vi "Weather Parse Test.vi"() -> ()   [LabVIEW 2020, in "CDM-Config.lvlib"]
uses:
  CDM-Config.lvlib
  <vilib>/httpClient/LabVIEWHTTPClient.lvlib
  Config-JSON/Config-JSON.lvclass
  Config Manager/Config Manager.lvclass
panel:
  out "error out":errorcluster
  in  "Tree":string(tree)
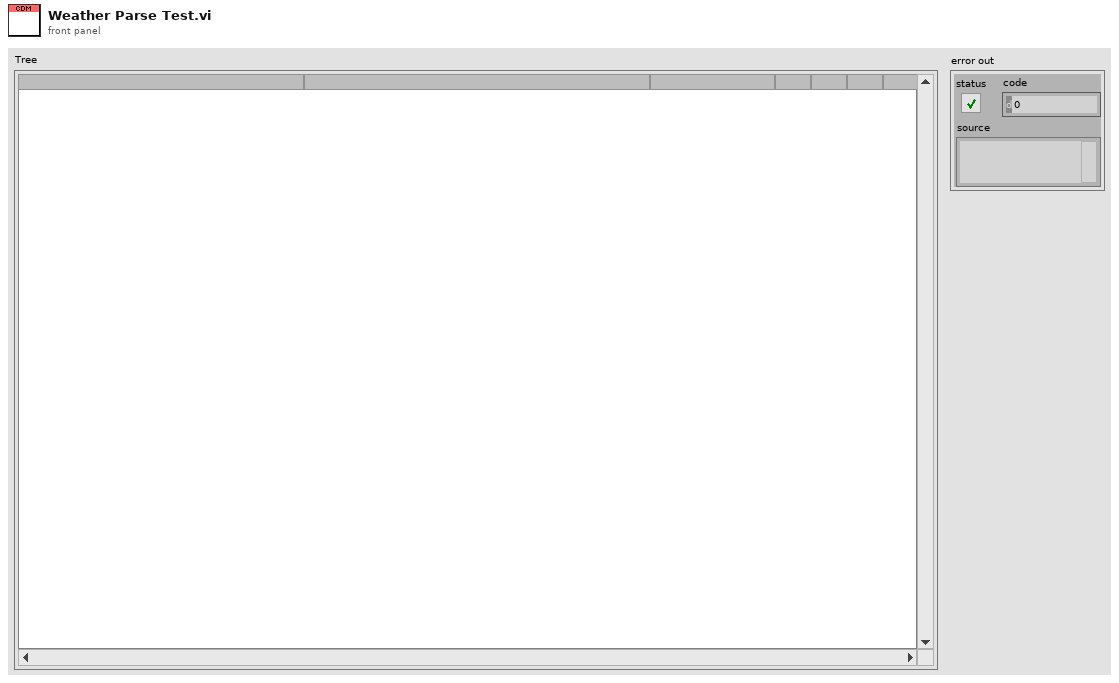
[diagram p1: front panel]
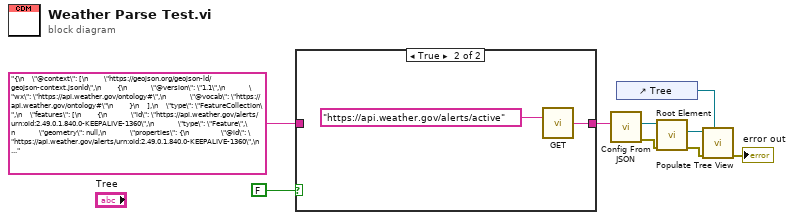
[diagram p0: block diagram]
diagram:
  n1 = case shown="True" FALSE {
    tunnel: [w10 w11] -> w7
    tunnel: "{\n    \"@context\": [\n        \"https://geojson.org/geojson-ld/geojson-context.jsonld\",\n        {\n            \"@version\": \"1.1\",\n            \"wx\": \"https://api.weather.gov/ontology#\",\n            \"@vocab\": \"https://api.weather.gov/ontology#\"\n        }\n    ],\n    \"type\": \"FeatureCollection\",\n    \"features\": [\n        {\n            \"id\": \"https://api.weather.gov/alerts/urn:oid:2.49.0.1.840.0-KEEPALIVE-1360\",\n            \"type\": \"Feature\",\n            \"geometry\": null,\n            \"properties\": {\n                \"@id\": \"https://api.weather.gov/alerts/urn:oid:2.49.0.1.840.0-KEEPALIVE-1360\",\n                \"@type\": \"wx:Alert\",\n                \"id\": \"urn:oid:2.49.0.1.840.0-KEEPALIVE-1360\",\n                \"areaDesc\": \"Montgomery\",\n                \"geocode\": {\n                    \"SAME\": [\n                        \"024031\"\n                    ],\n                    \"UGC\": [\n                        \"MDC031\"\n                    ]\n                },\n                \"affectedZones\": [\n                    \"https://api.weather.gov/zones/county/MDC031\"\n                ],\n                \"references\": [],\n                \"sent\": \"2025-12-03T16:14:45+00:00\",\n                \"effective\": \"2025-12-03T16:14:45+00:00\",\n                \"onset\": null,\n                \"expires\": \"2025-12-03T16:24:45+00:00\",\n                \"ends\": null,\n                \"status\": \"Test\",\n                \"messageType\": \"Alert\",\n                \"category\": \"Met\",\n                \"severity\": \"Unknown\",\n                \"certainty\": \"Unknown\",\n                \"urgency\": \"Unknown\",\n                \"event\": \"Test Message\",\n                \"sender\": \"w-nws.webmaster@noaa.gov\",\n                \"senderName\": \"NWS\",\n                \"headline\": null,\n                \"description\": \"Monitoring message only. Please disregard.\",\n                \"instruction\": \"Monitoring message only. Please disregard.\",\n                \"response\": \"None\",\n                \"parameters\": {\n                    \"AWIPSidentifier\": [\n                        \"KEPWBC\"\n                    ],\n                    \"WMOidentifier\": [\n                        \"NZUS91 KWBC 031614\"\n                    ],\n                    \"BLOCKCHANNEL\": [\n                        \"CMAS\",\n                        \"EAS\",\n                        \"NWEM\"\n                    ]\n                },\n                \"scope\": \"Public\",\n                \"code\": \"IPAWSv1.0\",\n                \"language\": \"en-US\",\n                \"web\": \"http://www.weather.gov\",\n                \"eventCode\": {\n                    \"SAME\": [\n                        \"NWS\"\n                    ],\n                    \"NationalWeatherService\": [\n                        \"TST\"\n                    ]\n                }\n            }\n        },\n        {\n            \"id\": \"https://api.weather.gov/alerts/urn:oid:2.49.0.1.840.0.cd44bbbaaabdcac51418f4171d6c2d57f83e8e62.002.1\",\n            \"type\": \"Feature\",\n            \"geometry\": null,\n            \"properties\": {\n                \"@id\": \"https://api.weather.gov/alerts/urn:oid:2.49.0.1.840.0.cd44bbbaaabdcac51418f4171d6c2d57f83e8e62.002.1\",\n                \"@type\": \"wx:Alert\",\n                \"id\": \"urn:oid:2.49.0.1.840.0.cd44bbbaaabdcac51418f4171d6c2d57f83e8e62.002.1\",\n                \"areaDesc\": \"Lake Michigan from Seul Choix Point to Rock Island Passage 5NM offshore to Mid Lake; Lake Michigan South of a line from Seul Choix Point to the Mackinac Bridge and North of a line from Charlevoix MI to South Fox Island 5NM offshore; Lake Michigan from Charlevoix to Point Betsie MI 5NM Offshore to mid lake; Lake Michigan from Point Betsie to Manistee MI 5NM offshore to Mid Lake; Lake Michigan from Rock Island Passage to Sturgeon Bay WI 5NM offshore to mid lake; Lake Michigan from Sturgeon Bay to Two Rivers WI 5NM offshore to Mid Lake\",\n                \"geocode\": {\n                    \"SAME\": [\n                        \"092261\",\n                        \"092362\",\n                        \"092364\",\n                        \"092366\",\n                        \"092563\",\n                        \"092565\"\n                    ],\n                    \"UGC\": [\n                        \"LMZ261\",\n                        \"LMZ362\",\n                        \"LMZ364\",\n                        \"LMZ366\",\n                        \"LMZ563\",\n                        \"LMZ565\"\n                    ]\n                },\n                \"affectedZones\": [\n                    \"https://api.weather.gov/zones/forecast/LMZ261\",\n                    \"https://api.weather.gov/zones/forecast/LMZ362\",\n                    \"https://api.weather.gov/zones/forecast/LMZ364\",\n                    \"https://api.weather.gov/zones/forecast/LMZ366\",\n                    \"https://api.weather.gov/zones/forecast/LMZ563\",\n                    \"https://api.weather.gov/zones/forecast/LMZ565\"\n                ],\n                \"references\": [\n                    {\n                        \"@id\": \"https://api.weather.gov/alerts/urn:oid:2.49.0.1.840.0.87140d8193f69fdde7a236498f0c417a3c416cc9.002.1\",\n                        \"identifier\": \"urn:oid:2.49.0.1.840.0.87140d8193f69fdde7a236498f0c417a3c416cc9.002.1\",\n                        \"sender\": \"w-nws.webmaster@noaa.gov\",\n                        \"sent\": \"2025-12-03T01:49:00-06:00\"\n                    }\n                ],\n                \"sent\": \"2025-12-03T10:07:00-06:00\",\n                \"effective\": \"2025-12-03T10:07:00-06:00\",\n                \"onset\": \"2025-12-04T21:00:00-06:00\",\n                \"expires\": \"2025-12-03T18:15:00-06:00\",\n                \"ends\": \"2025-12-05T06:00:00-06:00\",\n                \"status\": \"Actual\",\n                \"messageType\": \"Update\",\n                \"category\": \"Met\",\n                \"severity\": \"Moderate\",\n                \"certainty\": \"Possible\",\n                \"urgency\": \"Future\",\n                \"event\": \"Gale Watch\",\n                \"sender\": \"w-nws.webmaster@noaa.gov\",\n                \"senderName\": \"NWS Milwaukee/Sullivan WI\",\n                \"headline\": \"Gale Watch issued December 3 at 10:07AM CST until December 5 at 6:00AM CST by NWS Milwaukee/Sullivan WI\",\n                \"description\": \"* WHAT...Southwest winds 20 to 30 kt with gusts up to 40 kt and\\nwaves 7 to 12 ft possible.\\n\\n* WHERE...Northern Third of the Open Waters of Lake Michigan,\\nLake Michigan from Point Betsie to Manistee MI 5NM offshore to\\nMid Lake, and Lake Michigan from Sturgeon Bay to Two Rivers WI\\n5NM offshore to Mid Lake.\\n\\n* WHEN...From Thursday evening through late Thursday night.\\n\\n* IMPACTS...Strong winds can cause hazardous waves which could\\ncapsize or damage vessels and reduce visibility.\",\n                \"instruction\": \"Mariners should consider altering plans to avoid possible\\nhazardous conditions.  Remain in port, seek safe harbor, alter\\ncourse, and/or secure the vessel for severe wind and waves.\",\n                \"response\": \"Prepare\",\n                \"parameters\": {\n                    \"AWIPSidentifier\": [\n                        \"MWWMKX\"\n                    ],\n                    \"WMOidentifier\": [\n                        \"WHUS73 KMKX 031607\"\n                    ],\n                    \"NWSheadline\": [\n                        \"GALE WATCH REMAINS IN EFFECT FROM THURSDAY EVENING THROUGH LATE THURSDAY NIGHT\"\n                    ],\n                    \"BLOCKCHANNEL\": [\n                        \"EAS\",\n                        \"NWEM\",\n                        \"CMAS\"\n                    ],\n                    \"VTEC\": [\n                        \"/O.CON.KMKX.GL.A.0026.251205T0300Z-251205T1200Z/\"\n                    ],\n                    \"eventEndingTime\": [\n                        \"2025-12-05T06:00:00-06:00\"\n                    ]\n                },\n                \"scope\": \"Public\",\n                \"code\": \"IPAWSv1.0\",\n                \"language\": \"en-US\",\n                \"web\": \"http://www.weather.gov\",\n                \"eventCode\": {\n                    \"SAME\": [\n                        \"NWS\"\n                    ],\n                    \"NationalWeatherService\": [\n                        \"GLA\"\n                    ]\n                }\n            }\n        },\n        {\n            \"id\": \"https://api.weather.gov/alerts/urn:oid:2.49.0.1.840.0.cd44bbbaaabdcac51418f4171d6c2d57f83e8e62.001.1\",\n            \"type\": \"Feature\",\n            \"geometry\": null,\n            \"properties\": {\n                \"@id\": \"https://api.weather.gov/alerts/urn:oid:2.49.0.1.840.0.cd44bbbaaabdcac51418f4171d6c2d57f83e8e62.001.1\",\n                \"@type\": \"wx:Alert\",\n                \"id\": \"urn:oid:2.49.0.1.840.0.cd44bbbaaabdcac51418f4171d6c2d57f83e8e62.001.1\",\n                \"areaDesc\": \"Sheboygan to Port Washington WI; Port Washington to North Point Light WI; North Point Light to Wind Point WI; Wind Point WI to Winthrop Harbor IL\",\n                \"geocode\": {\n                    \"SAME\": [\n                        \"092643\",\n                        \"092644\",\n                        \"092645\",\n                        \"092646\"\n                    ],\n                    \"UGC\": [\n                        \"LMZ643\",\n                        \"LMZ644\",\n                        \"LMZ645\",\n                        \"LMZ646\"\n                    ]\n                },\n                \"affectedZones\": [\n                    \"https://api.weather.gov/zones/forecast/LMZ643\",\n                    \"https://api.weather.gov/zones/forecast/LMZ644\",\n                    \"https://api.weather.gov/zones/forecast/LMZ645\",\n                    \"https://api.weather.gov/zones/forecast/LMZ646\"\n                ],\n                \"references\": [\n                    {\n                        \"@id\": \"https://api.weather.gov/alerts/urn:oid:2.49.0.1.840.0.87140d8193f69fdde7a236498f0c417a3c416cc9.001.1\",\n                        \"identifier\": \"urn:oid:2.49.0.1.840.0.87140d8193f69fdde7a236498f0c417a3c416cc9.001.1\",\n                        \"sender\": \"w-nws.webmaster@noaa.gov\",\n                        \"sent\": \"2025-12-03T01:49:00-06:00\"\n                    }\n                ],\n                \"sent\": \"2025-12-03T10:07:00-06:00\",\n                \"effective\": \"2025-12-03T10:07:00-06:00\",\n                \"onset\": \"2025-12-03T10:07:00-06:00\",\n                \"expires\": \"2025-12-03T18:15:00-06:00\",\n                \"ends\": \"2025-12-04T06:00:00-06:00\",\n                \"status\": \"Actual\",\n                \"messageType\": \"Update\",\n                \"category\": \"Met\",\n                \"severity\": \"Minor\",\n                \"certainty\": \"Likely\",\n                \"urgency\": \"Expected\",\n                \"event\": \"Small Craft Advisory\",\n                \"sender\": \"w-nws.webmaster@noaa.gov\",\n                \"senderName\": \"NWS Milwaukee/Sullivan WI\",\n                \"headline\": \"Small Craft Advisory issued December 3 at 10:07AM CST until December 4 at 6:00AM CST by NWS Milwaukee/Sullivan WI\",\n                \"description\": \"* WHAT...Northwest winds 15 to 20 kt with gusts up to 25 kt.\\n\\n* WHERE...Nearshore Waters from Sheboygan to Winthrop Harbor IL.\\n\\n* WHEN...Until 6 AM CST Thursday.\\n\\n* IMPACTS...Conditions will be hazardous to small craft.\",\n                \"instruction\": \"Inexperienced mariners, especially those operating smaller\\nvessels, should avoid navigating in hazardous conditions.\",\n                \"response\": \"Avoid\",\n                \"parameters\": {\n                    \"AWIPSidentifier\": [\n                        \"MWWMKX\"\n                    ],\n                    \"WMOidentifier\": [\n                        \"WHUS73 KMKX 031607\"\n                    ],\n                    \"NWSheadline\": [\n                        \"SMALL CRAFT ADVISORY REMAINS IN EFFECT UNTIL 6 AM CST THURSDAY\"\n                    ],\n                    \"BLOCKCHANNEL\": [\n                        \"EAS\",\n                        \"NWEM\",\n                        \"CMAS\"\n                    ],\n                    \"VTEC\": [\n                        \"/O.CON.KMKX.SC.Y.0105.000000T0000Z-251204T1200Z/\"\n                    ],\n                    \"eventEndingTime\": [\n                        \"2025-12-04T06:00:00-06:00\"\n                    ],\n                    \"expiredReferences\": [\n                        \"w-nws.webmaster@noaa.gov,urn:oid:2.49.0.1.840.0.8bd0308a1f57db3dacad4c3397c13ff936336f9a.001.1,2025-12-02T20:55:00-06:00 w-nws.webmaster@noaa.gov,urn:oid:2.49.0.1.840.0.6281cc536b0e67be3da54b18c0c55c2862a1bde1.001.1,2025-12-02T14:15:00-06:00 w-nws.webmaster@noaa.gov,urn:oid:2.49.0.1.840.0.2f172b9f18f65013fb5f156b8abb524ff0d234b7.001.1,2025-12-02T08:57:00-06:00 w-nws.webmaster@noaa.gov,urn:oid:2.49.0.1.840.0.b1896b6562e7fd8378f844b86b23eedf120466cc.001.1,2025-12-02T02:26:00-06:00\"\n                    ]\n                },\n                \"scope\": \"Public\",\n                \"code\": \"IPAWSv1.0\",\n                \"language\": \"en-US\",\n                \"web\": \"http://www.weather.gov\",\n                \"eventCode\": {\n                    \"SAME\": [\n                        \"NWS\"\n                    ],\n                    \"NationalWeatherService\": [\n                        \"SCY\"\n                    ]\n                }\n            }\n        },\n        {\n            \"id\": \"https://api.weather.gov/alerts/urn:oid:2.49.0.1.840.0.cfec64fd36b2ac790d0ebe73b8c20f8dfc3ec5cb.007.1\",\n            \"type\": \"Feature\",\n            \"geometry\": null,\n            \"properties\": {\n                \"@id\": \"https://api.weather.gov/alerts/urn:oid:2.49.0.1.840.0.cfec64fd36b2ac790d0ebe73b8c20f8dfc3ec5cb.007.1\",\n                \"@type\": \"wx:Alert\",\n                \"id\": \"urn:oid:2.49.0.1.840.0.cfec64fd36b2ac790d0ebe73b8c20f8dfc3ec5cb.007.1\",\n                \"areaDesc\": \"Saxon Harbor WI to Black River MI\",\n                \"geocode\": {\n                    \"SAME\": [\n                        \"091240\"\n                    ],\n                    \"UGC\": [\n                        \"LSZ240\"\n                    ]\n                },\n                \"affectedZones\": [\n                    \"https://api.weather.gov/zones/forecast/LSZ240\"\n                ],\n                \"references\": [\n                    {\n                        \"@id\": \"https://api.weather.gov/alerts/urn:oid:2.49.0.1.840.0.e016f252f56054b547b3ac73b3419f6e51da412e.009.1\",\n                        \"identifier\": \"urn:oid:2.49.0.1.840.0.e016f252f56054b547b3ac73b3419f6e51da412e.009.1\",\n                        \"sender\": \"w-nws.webmaster@noaa.gov\",\n                        \"sent\": \"2025-12-03T03:23:00-05:00\"\n                    }\n                ],\n                \"sent\": \"2025-12-03T10:58:00-05:00\",\n                \"effective\": \"2025-12-03T10:58:00-05:00\",\n                \"onset\": \"2025-12-03T10:58:00-05:00\",\n                \"expires\": \"2025-12-03T23:00:00-05:00\",\n                \"ends\": \"2025-12-04T07:00:00-05:00\",\n                \"status\": \"Actual\",\n                \"messageType\": \"Update\",\n                \"category\": \"Met\",\n                \"severity\": \"Minor\",\n                \"certainty\": \"Likely\",\n                \"urgency\": \"Expected\",\n                \"event\": \"Small Craft Advisory\",\n                \"sender\": \"w-nws.webmaster@noaa.gov\",\n                \"senderName\": \"NWS Marquette MI\",\n                \"headline\": \"Small Craft Advisory issued December 3 at 10:58AM EST until December 4 at 7:00AM EST by NWS Marquette MI\",\n                \"description\": \"* WHAT...Northwest winds 15 to 25 kt with gusts up to 30 kt and\\nwaves 4 to 7 ft occurring.\\n\\n* WHERE...Saxon Harbor WI to Black River MI.\\n\\n* WHEN...Until 7 AM EST /6 AM CST/ Thursday.\\n\\n* IMPACTS...Conditions will be hazardous to small craft.\",\n                \"instruction\": \"Inexperienced mariners, especially those operating smaller\\nvessels, should avoid navigating in hazardous conditions.\",\n                \"response\": \"Avoid\",\n                \"parameters\": {\n                    \"AWIPSidentifier\": [\n                        \"MWWMQT\"\n                    ],\n                    \"WMOidentifier\": [\n                        \"WHUS73 KMQT 031558\"\n                    ],\n                    \"NWSheadline\": [\n                        \"SMALL CRAFT ADVISORY REMAINS IN EFFECT UNTIL 7 AM EST /6 AM CST/ THURSDAY\"\n                    ],\n                    \"BLOCKCHANNEL\": [\n                        \"EAS\",\n                        \"NWEM\",\n                        \"CMAS\"\n                    ],\n                    \"VTEC\": [\n                        \"/O.CON.KMQT.SC.Y.0191.000000T0000Z-251204T1200Z/\"\n                    ],\n                    \"eventEndingTime\": [\n                        \"2025-12-04T07:00:00-05:00\"\n                    ],\n                    \"expiredReferences\": [\n                        \"w-nws.webmaster@noaa.gov,urn:oid:2.49.0.1.840.0.012a713e44cf33f321dde7a7dd606454111e7dbb.005.1,2025-12-02T22:29:00-05:00 w-nws.webmaster@noaa.gov,urn:oid:2.49.0.1.840.0.74d44099106d0ecd40f7d2a62c56231069593ff3.005.1,2025-12-02T14:53:00-05:00 w-nws.webmaster@noaa.gov,urn:oid:2.49.0.1.840.0.747dd730e6a8b18ac9024c3c055a74162144c3ca.001.1,2025-12-02T10:16:00-05:00 w-nws.webmaster@noaa.gov,urn:oid:2.49.0.1.840.0.9d4c1194cc60ce916e8ebdf8581f4113872ed30b.001.1,2025-12-02T03:21:00-05:00\"\n                    ]\n                },\n                \"scope\": \"Public\",\n                \"code\": \"IPAWSv1.0\",\n                \"language\": \"en-US\",\n                \"web\": \"http://www.weather.gov\",\n                \"eventCode\": {\n                    \"SAME\": [\n                        \"NWS\"\n                    ],\n                    \"NationalWeatherService\": [\n                        \"SCY\"\n                    ]\n                }\n            }\n        },\n        {\n            \"id\": \"https://api.weather.gov/alerts/urn:oid:2.49.0.1.840.0.cfec64fd36b2ac790d0ebe73b8c20f8dfc3ec5cb.005.1\",\n            \"type\": \"Feature\",\n            \"geometry\": null,\n            \"properties\": {\n                \"@id\": \"https://api.weather.gov/alerts/urn:oid:2.49.0.1.840.0.cfec64fd36b2ac790d0ebe73b8c20f8dfc3ec5cb.005.1\",\n                \"@type\": \"wx:Alert\",\n                \"id\": \"urn:oid:2.49.0.1.840.0.cfec64fd36b2ac790d0ebe73b8c20f8dfc3ec5cb.005.1\",\n                \"areaDesc\": \"Upper Entrance of Portage Canal to Eagle River MI; Manitou Island to Point Isabelle MI; Point Isabelle to Lower Entrance of Portage Canal MI; Portage Lake to Huron Island MI to Lower Entrance of Portage Canal To Huron Islands MI Including Keweenaw and Huron Bays; Huron Islands to Marquette MI; Marquette to Munising MI; Munising to Grand Marais MI; Grand Marais to Whitefish Point MI; Lake Superior West of Line from Manitou Island to Marquette MI Beyond 5NM from shore; Lake Superior from Grand Marais MI to Whitefish Point MI 5NM off shore to the US/Canadian border\",\n                \"geocode\": {\n                    \"SAME\": [\n                        \"091243\",\n                        \"091245\",\n                        \"091246\",\n                        \"091247\",\n                        \"091248\",\n                        \"091249\",\n                        \"091250\",\n                        \"091251\",\n                        \"091265\",\n                        \"091267\"\n                    ],\n                    \"UGC\": [\n                        \"LSZ243\",\n                        \"LSZ245\",\n                        \"LSZ246\",\n                        \"LSZ247\",\n                        \"LSZ248\",\n                        \"LSZ249\",\n                        \"LSZ250\",\n                        \"LSZ251\",\n                        \"LSZ265\",\n                        \"LSZ267\"\n                    ]\n                },\n                \"affectedZones\": [\n                    \"https://api.weather.gov/zones/forecast/LSZ243\",\n                    \"https://api.weather.gov/zones/forecast/LSZ245\",\n                    \"https://api.weather.gov/zones/forecast/LSZ246\",\n                    \"https://api.weather.gov/zones/forecast/LSZ247\",\n                    \"https://api.weather.gov/zones/forecast/LSZ248\",\n                    \"https://api.weather.gov/zones/forecast/LSZ249\",\n                    \"https://api.weather.gov/zones/forecast/LSZ250\",\n                    \"https://api.weather.gov/zones/forecast/LSZ251\",\n                    \"https://api.weather.gov/zones/forecast/LSZ265\",\n                    \"https://api.weather.gov/zones/forecast/LSZ267\"\n                ],\n                \"references\": [\n                    {\n                        \"@id\": \"https://api.weather.gov/alerts/urn:oid:2.49.0.1.840.0.e016f252f56054b547b3ac73b3419f6e51da412e.006.3\",\n                        \"identifier\": \"urn:oid:2.49.0.1.840.0.e016f252f56054b547b3ac73b3419f6e51da412e.006.3\",\n                        \"sender\": \"w-nws.webmaster@noaa.gov\",\n                        \"sent\": \"2025-12-03T03:23:00-05:00\"\n                    },\n                    {\n                        \"@id\": \"https://api.weather.gov/alerts/urn:oid:2.49.0.1.840.0.e016f252f56054b547b3ac73b3419f6e51da412e.007.3\",\n                        \"identifier\": \"urn:oid:2.49.0.1.840.0.e016f252f56054b547b3ac73b3419f6e51da412e.007.3\",\n                        \"sender\": \"w-nws.webmaster@noaa.gov\",\n                        \"sent\": \"2025-12-03T03:23:00-05:00\"\n                    },\n                    {\n                        \"@id\": \"https://api.weather.gov/alerts/urn:oid:2.49.0.1.840.0.e016f252f56054b547b3ac73b3419f6e51da412e.008.2\",\n                        \"identifier\": \"urn:oid:2.49.0.1.840.0.e016f252f56054b547b3ac73b3419f6e51da412e.008.2\",\n                        \"sender\": \"w-nws.webmaster@noaa.gov\",\n                        \"sent\": \"2025-12-03T03:23:00-05:00\"\n                    }\n                ],\n                \"sent\": \"2025-12-03T10:58:00-05:00\",\n                \"effective\": \"2025-12-03T10:58:00-05:00\",\n                \"onset\": \"2025-12-03T10:58:00-05:00\",\n                \"expires\": \"2025-12-03T23:00:00-05:00\",\n                \"ends\": \"2025-12-04T07:00:00-05:00\",\n                \"status\": \"Actual\",\n                \"messageType\": \"Update\",\n                \"category\": \"Met\",\n                \"severity\": \"Moderate\",\n                \"certainty\": \"Likely\",\n                \"urgency\": \"Expected\",\n                \"event\": \"Gale Warning\",\n                \"sender\": \"w-nws.webmaster@noaa.gov\",\n                \"senderName\": \"NWS Marquette MI\",\n                \"headline\": \"Gale Warning issued December 3 at 10:58AM EST until December 4 at 7:00AM EST by NWS Marquette MI\",\n                \"description\": \"* WHAT...Northwest winds 20 to 30 kt with gusts up to 35 kt and\\nwaves 8 to 13 ft occurring.\\n\\n* WHERE...Portions of Central, Eastern and Western Lake Superior.\\n\\n* WHEN...Until 7 AM EST Thursday.\\n\\n* IMPACTS...Strong winds will cause hazardous waves which could\\ncapsize or damage vessels and reduce visibility.\",\n                \"instruction\": \"Mariners should alter plans to avoid these hazardous conditions.\\nRemain in port, seek safe harbor, alter course, and/or secure the\\nvessel for hazardous conditions.\",\n                \"response\": \"Avoid\",\n                \"parameters\": {\n                    \"AWIPSidentifier\": [\n                        \"MWWMQT\"\n                    ],\n                    \"WMOidentifier\": [\n                        \"WHUS73 KMQT 031558\"\n                    ],\n                    \"NWSheadline\": [\n                        \"GALE WARNING REMAINS IN EFFECT UNTIL 7 AM EST THURSDAY\"\n                    ],\n                    \"BLOCKCHANNEL\": [\n                        \"EAS\",\n                        \"NWEM\",\n                        \"CMAS\"\n                    ],\n                    \"VTEC\": [\n                        \"/O.CON.KMQT.GL.W.0057.000000T0000Z-251204T1200Z/\"\n                    ],\n                    \"eventEndingTime\": [\n                        \"2025-12-04T07:00:00-05:00\"\n                    ]\n                },\n                \"scope\": \"Public\",\n                \"code\": \"IPAWSv1.0\",\n                \"language\": \"en-US\",\n                \"web\": \"http://www.weather.gov\",\n                \"eventCode\": {\n                    \"SAME\": [\n                        \"NWS\"\n                    ],\n                    \"NationalWeatherService\": [\n                        \"GLW\"\n                    ]\n                }\n            }\n        },\n        {\n            \"id\": \"https://api.weather.gov/alerts/urn:oid:2.49.0.1.840.0.cfec64fd36b2ac790d0ebe73b8c20f8dfc3ec5cb.001.1\",\n            \"type\": \"Feature\",\n            \"geometry\": null,\n            \"properties\": {\n                \"@id\": \"https://api.weather.gov/alerts/urn:oid:2.49.0.1.840.0.cfec64fd36b2ac790d0ebe73b8c20f8dfc3ec5cb.001.1\",\n                \"@type\": \"wx:Alert\",\n                \"id\": \"urn:oid:2.49.0.1.840.0.cfec64fd36b2ac790d0ebe73b8c20f8dfc3ec5cb.001.1\",\n                \"areaDesc\": \"Eagle River to Manitou Island MI; Lake Superior from Upper Entrance to Portage Canal to Manitou Island MI 5NM off shore to the US/Canadian Border; Lake Superior East of a line from Manitou Island to Marquette MI and West of a line from Grand Marais MI to the US/Canadian Border Beyond 5NM from shore\",\n                \"geocode\": {\n                    \"SAME\": [\n                        \"091244\",\n                        \"091264\",\n                        \"091266\"\n                    ],\n                    \"UGC\": [\n                        \"LSZ244\",\n                        \"LSZ264\",\n                        \"LSZ266\"\n                    ]\n                },\n                \"affectedZones\": [\n                    \"https://api.weather.gov/zones/forecast/LSZ244\",\n                    \"https://api.weather.gov/zones/forecast/LSZ264\",\n                    \"https://api.weather.gov/zones/forecast/LSZ266\"\n                ],\n                \"references\": [\n                    {\n                        \"@id\": \"https://api.weather.gov/alerts/urn:oid:2.49.0.1.840.0.e016f252f56054b547b3ac73b3419f6e51da412e.001.3\",\n                        \"identifier\": \"urn:oid:2.49.0.1.840.0.e016f252f56054b547b3ac73b3419f6e51da412e.001.3\",\n                        \"sender\": \"w-nws.webmaster@noaa.gov\",\n                        \"sent\": \"2025-12-03T03:23:00-05:00\"\n                    },\n                    {\n                        \"@id\": \"https://api.weather.gov/alerts/urn:oid:2.49.0.1.840.0.e016f252f56054b547b3ac73b3419f6e51da412e.003.2\",\n                        \"identifier\": \"urn:oid:2.49.0.1.840.0.e016f252f56054b547b3ac73b3419f6e51da412e.003.2\",\n                        \"sender\": \"w-nws.webmaster@noaa.gov\",\n                        \"sent\": \"2025-12-03T03:23:00-05:00\"\n                    }\n                ],\n                \"sent\": \"2025-12-03T10:58:00-05:00\",\n                \"effective\": \"2025-12-03T10:58:00-05:00\",\n                \"onset\": \"2025-12-03T10:58:00-05:00\",\n                \"expires\": \"2025-12-03T23:00:00-05:00\",\n                \"ends\": \"2025-12-04T07:00:00-05:00\",\n                \"status\": \"Actual\",\n                \"messageType\": \"Update\",\n                \"category\": \"Met\",\n                \"severity\": \"Moderate\",\n                \"certainty\": \"Likely\",\n                \"urgency\": \"Expected\",\n                \"event\": \"Gale Warning\",\n                \"sender\": \"w-nws.webmaster@noaa.gov\",\n                \"senderName\": \"NWS Marquette MI\",\n                \"headline\": \"Gale Warning issued December 3 at 10:58AM EST until December 4 at 7:00AM EST by NWS Marquette MI\",\n                \"description\": \"* WHAT...For the Gale Warning, northwest winds 25 to 30 kt with\\ngusts up to 40 kt and waves 8 to 13 ft occurring. For the\\nHeavy Freezing Spray Warning, heavy freezing spray at a rate\\nof 2 cm per hour or greater expected, and may rapidly\\naccumulate on vessels.\\n\\n* WHERE...Eagle River to Manitou Island MI, Lake Superior from\\nUpper Entrance to Portage Canal to Manitou Island MI 5NM off\\nshore to the US/Canadian Border and Lake Superior East of a\\nline from Manitou Island to Marquette MI and West of a line\\nfrom Grand Marais MI to the US/Canadian Border Beyond 5NM from\\nshore.\\n\\n* WHEN...For the Gale Warning, until 7 AM EST Thursday. For the\\nHeavy Freezing Spray Warning, from 7 PM this evening to 7 AM\\nEST Thursday.\\n\\n* IMPACTS...Operating a vessel in heavy freezing spray is\\nhazardous. Freezing spray may render mechanical and electronic\\ncomponents inoperative. Rapid ice accretion on decks and\\nsuperstructures may result in a catastrophic loss of\\nstability. Strong winds will cause hazardous waves which could\\ncapsize or damage vessels and reduce visibility.\",\n                \"instruction\": \"Mariners should prepare for dangerous accumulation of ice on\\ntheir vessel. If possible, remain in port, avoid the warning area\\nor conduct mitigation.\\n\\nMariners should alter plans to avoid these hazardous conditions.\\nRemain in port, seek safe harbor, alter course, and/or secure the\\nvessel for hazardous conditions.\",\n                \"response\": \"Avoid\",\n                \"parameters\": {\n                    \"AWIPSidentifier\": [\n                        \"MWWMQT\"\n                    ],\n                    \"WMOidentifier\": [\n                        \"WHUS73 KMQT 031558\"\n                    ],\n                    \"NWSheadline\": [\n                        \"GALE WARNING REMAINS IN EFFECT UNTIL 7 AM EST THURSDAY... ...HEAVY FREEZING SPRAY WARNING REMAINS IN EFFECT FROM 7 PM THIS EVENING TO 7 AM EST THURSDAY\"\n                    ],\n                    \"BLOCKCHANNEL\": [\n                        \"EAS\",\n                        \"NWEM\",\n                        \"CMAS\"\n                    ],\n                    \"VTEC\": [\n                        \"/O.CON.KMQT.GL.W.0057.000000T0000Z-251204T1200Z/\"\n                    ],\n                    \"eventEndingTime\": [\n                        \"2025-12-04T07:00:00-05:00\"\n                    ]\n                },\n                \"scope\": \"Public\",\n                \"code\": \"IPAWSv1.0\",\n                \"language\": \"en-US\",\n                \"web\": \"http://www.weather.gov\",\n                \"eventCode\": {\n                    \"SAME\": [\n                        \"NWS\"\n                    ],\n                    \"NationalWeatherService\": [\n                        \"GLW\"\n                    ]\n                }\n            }\n        },\n        {\n            \"id\": \"https://api.weather.gov/alerts/urn:oid:2.49.0.1.840.0.cfec64fd36b2ac790d0ebe73b8c20f8dfc3ec5cb.006.2\",\n            \"type\": \"Feature\",\n            \"geometry\": null,\n            \"properties\": {\n                \"@id\": \"https://api.weather.gov/alerts/urn:oid:2.49.0.1.840.0.cfec64fd36b2ac790d0ebe73b8c20f8dfc3ec5cb.006.2\",\n                \"@type\": \"wx:Alert\",\n                \"id\": \"urn:oid:2.49.0.1.840.0.cfec64fd36b2ac790d0ebe73b8c20f8dfc3ec5cb.006.2\",\n                \"areaDesc\": \"Green Bay North of line from Cedar River MI to Rock Island Passage; Seul Choix Point to Point Detour MI; 5NM East of a line from Fairport MI to Rock Island Passage\",\n                \"geocode\": {\n                    \"SAME\": [\n                        \"092221\",\n                        \"092248\",\n                        \"092250\"\n                    ],\n                    \"UGC\": [\n                        \"LMZ221\",\n                        \"LMZ248\",\n                        \"LMZ250\"\n                    ]\n                },\n                \"affectedZones\": [\n                    \"https://api.weather.gov/zones/forecast/LMZ221\",\n                    \"https://api.weather.gov/zones/forecast/LMZ248\",\n                    \"https://api.weather.gov/zones/forecast/LMZ250\"\n                ],\n                \"references\": [\n                    {\n                        \"@id\": \"https://api.weather.gov/alerts/urn:oid:2.49.0.1.840.0.e016f252f56054b547b3ac73b3419f6e51da412e.010.2\",\n                        \"identifier\": \"urn:oid:2.49.0.1.840.0.e016f252f56054b547b3ac73b3419f6e51da412e.010.2\",\n                        \"sender\": \"w-nws.webmaster@noaa.gov\",\n                        \"sent\": \"2025-12-03T03:23:00-05:00\"\n                    }\n                ],\n                \"sent\": \"2025-12-03T10:58:00-05:00\",\n                \"effective\": \"2025-12-03T10:58:00-05:00\",\n                \"onset\": \"2025-12-04T22:00:00-05:00\",\n                \"expires\": \"2025-12-03T23:00:00-05:00\",\n                \"ends\": \"2025-12-05T07:00:00-05:00\",\n                \"status\": \"Actual\",\n                \"messageType\": \"Update\",\n                \"category\": \"Met\",\n                \"severity\": \"Moderate\",\n                \"certainty\": \"Possible\",\n                \"urgency\": \"Future\",\n                \"event\": \"Gale Watch\",\n                \"sender\": \"w-nws.webmaster@noaa.gov\",\n                \"senderName\": \"NWS Marquette MI\",\n                \"headline\": \"Gale Watch issued December 3 at 10:58AM EST until December 5 at 7:00AM EST by NWS Marquette MI\",\n                \"description\": \"* WHAT...For the Small Craft Advisory, northwest winds 15 to 25\\nkt with gusts up to 30 kt and waves 1 to 4 ft occurring. For\\nthe Gale Watch, southwest winds 20 to 30 kt with gusts up to\\n35 kt and waves 5 to 8 ft possible.\\n\\n* WHERE...Green Bay North of line from Cedar River MI to Rock\\nIsland Passage, Seul Choix Point to Point Detour MI and 5NM\\nEast of a line from Fairport MI to Rock Island Passage.\\n\\n* WHEN...For the Small Craft Advisory, until 7 AM EST Thursday.\\nFor the Gale Watch, from Thursday evening through Friday\\nmorning.\\n\\n* IMPACTS...Strong winds can cause hazardous waves which could\\ncapsize or damage vessels and reduce visibility.\",\n                \"instruction\": \"Mariners should consider altering plans to avoid possible\\nhazardous conditions.  Remain in port, seek safe harbor, alter\\ncourse, and/or secure the vessel for severe wind and waves.\",\n                \"response\": \"Prepare\",\n                \"parameters\": {\n                    \"AWIPSidentifier\": [\n                        \"MWWMQT\"\n                    ],\n                    \"WMOidentifier\": [\n                        \"WHUS73 KMQT 031558\"\n                    ],\n                    \"NWSheadline\": [\n                        \"SMALL CRAFT ADVISORY REMAINS IN EFFECT UNTIL 7 AM EST THURSDAY... ...GALE WATCH REMAINS IN EFFECT FROM THURSDAY EVENING THROUGH FRIDAY MORNING\"\n                    ],\n                    \"BLOCKCHANNEL\": [\n                        \"EAS\",\n                        \"NWEM\",\n                        \"CMAS\"\n                    ],\n                    \"VTEC\": [\n                        \"/O.CON.KMQT.GL.A.0034.251205T0300Z-251205T1200Z/\"\n                    ],\n                    \"eventEndingTime\": [\n                        \"2025-12-05T07:00:00-05:00\"\n                    ]\n                },\n                \"scope\": \"Public\",\n                \"code\": \"IPAWSv1.0\",\n                \"language\": \"en-US\",\n                \"web\": \"http://www.weather.gov\",\n                \"eventCode\": {\n                    \"SAME\": [\n                        \"NWS\"\n                    ],\n                    \"NationalWeatherService\": [\n                        \"GLA\"\n                    ]\n                }\n            }\n        },\n        {\n            \"id\": \"https://api.weather.gov/alerts/urn:oid:2.49.0.1.840.0.cfec64fd36b2ac790d0ebe73b8c20f8dfc3ec5cb.004.2\",\n            \"type\": \"Feature\",\n            \"geometry\": null,\n            \"properties\": {\n                \"@id\": \"https://api.weather.gov/alerts/urn:oid:2.49.0.1.840.0.cfec64fd36b2ac790d0ebe73b8c20f8dfc3ec5cb.004.2\",\n                \"@type\": \"wx:Alert\",\n                \"id\": \"urn:oid:2.49.0.1.840.0.cfec64fd36b2ac790d0ebe73b8c20f8dfc3ec5cb.004.2\",\n                \"areaDesc\": \"Ontonagon to Upper Entrance of Portage Canal MI\",\n                \"geocode\": {\n                    \"SAME\": [\n                        \"091242\"\n                    ],\n                    \"UGC\": [\n                        \"LSZ242\"\n                    ]\n                },\n                \"affectedZones\": [\n                    \"https://api.weather.gov/zones/forecast/LSZ242\"\n                ],\n                \"references\": [\n                    {\n                        \"@id\": \"https://api.weather.gov/alerts/urn:oid:2.49.0.1.840.0.e016f252f56054b547b3ac73b3419f6e51da412e.005.3\",\n                        \"identifier\": \"urn:oid:2.49.0.1.840.0.e016f252f56054b547b3ac73b3419f6e51da412e.005.3\",\n                        \"sender\": \"w-nws.webmaster@noaa.gov\",\n                        \"sent\": \"2025-12-03T03:23:00-05:00\"\n                    }\n                ],\n                \"sent\": \"2025-12-03T10:58:00-05:00\",\n                \"effective\": \"2025-12-03T10:58:00-05:00\",\n                \"onset\": \"2025-12-03T16:00:00-05:00\",\n                \"expires\": \"2025-12-03T23:00:00-05:00\",\n                \"ends\": \"2025-12-04T01:00:00-05:00\",\n                \"status\": \"Actual\",\n                \"messageType\": \"Update\",\n                \"category\": \"Met\",\n                \"severity\": \"Moderate\",\n                \"certainty\": \"Likely\",\n                \"urgency\": \"Expected\",\n                \"event\": \"Gale Warning\",\n                \"sender\": \"w-nws.webmaster@noaa.gov\",\n                \"senderName\": \"NWS Marquette MI\",\n                \"headline\": \"Gale Warning issued December 3 at 10:58AM EST until December 4 at 1:00AM EST by NWS Marquette MI\",\n                \"description\": \"* WHAT...For the Small Craft Advisory, northwest winds 20 to 25\\nkt with gusts up to 30 kt and waves 6 to 8 ft occurring. For\\nthe Gale Warning, northwest winds 20 to 30 kt with gusts up to\\n35 kt and waves 7 to 10 ft expected.\\n\\n* WHERE...Ontonagon to Upper Entrance of Portage Canal MI.\\n\\n* WHEN...For the Small Craft Advisory, until 4 PM EST this\\nafternoon. For the Gale Warning, from 4 PM this afternoon to 1\\nAM EST Thursday.\\n\\n* IMPACTS...Strong winds will cause hazardous waves which could\\ncapsize or damage vessels and reduce visibility.\",\n                \"instruction\": \"Mariners should alter plans to avoid these hazardous conditions.\\nRemain in port, seek safe harbor, alter course, and/or secure the\\nvessel for hazardous conditions.\",\n                \"response\": \"Avoid\",\n                \"parameters\": {\n                    \"AWIPSidentifier\": [\n                        \"MWWMQT\"\n                    ],\n                    \"WMOidentifier\": [\n                        \"WHUS73 KMQT 031558\"\n                    ],\n                    \"NWSheadline\": [\n                        \"SMALL CRAFT ADVISORY REMAINS IN EFFECT UNTIL 4 PM EST THIS AFTERNOON... ...GALE WARNING REMAINS IN EFFECT FROM 4 PM THIS AFTERNOON TO 1 AM EST THURSDAY\"\n                    ],\n                    \"BLOCKCHANNEL\": [\n                        \"EAS\",\n                        \"NWEM\",\n                        \"CMAS\"\n                    ],\n                    \"VTEC\": [\n                        \"/O.CON.KMQT.GL.W.0057.251203T2100Z-251204T0600Z/\"\n                    ],\n                    \"eventEndingTime\": [\n                        \"2025-12-04T01:00:00-05:00\"\n                    ]\n                },\n                \"scope\": \"Public\",\n                \"code\": \"IPAWSv1.0\",\n                \"language\": \"en-US\",\n                \"web\": \"http://www.weather.gov\",\n                \"eventCode\": {\n                    \"SAME\": [\n                        \"NWS\"\n                    ],\n                    \"NationalWeatherService\": [\n                        \"GLW\"\n                    ]\n                }\n            }\n        },\n        {\n            \"id\": \"https://api.weather.gov/alerts/urn:oid:2.49.0.1.840.0.cfec64fd36b2ac790d0ebe73b8c20f8dfc3ec5cb.002.1\",\n            \"type\": \"Feature\",\n            \"geometry\": null,\n            \"properties\": {\n                \"@id\": \"https://api.weather.gov/alerts/urn:oid:2.49.0.1.840.0.cfec64fd36b2ac790d0ebe73b8c20f8dfc3ec5cb.002.1\",\n                \"@type\": \"wx:Alert\",\n                \"id\": \"urn:oid:2.49.0.1.840.0.cfec64fd36b2ac790d0ebe73b8c20f8dfc3ec5cb.002.1\",\n                \"areaDesc\": \"Lake Superior from Saxon Harbor WI to Upper Entrance to Portage Canal MI 5NM off shore to the US/Canadian border including Isle Royale National Park\",\n                \"geocode\": {\n                    \"SAME\": [\n                        \"091263\"\n                    ],\n                    \"UGC\": [\n                        \"LSZ263\"\n                    ]\n                },\n                \"affectedZones\": [\n                    \"https://api.weather.gov/zones/forecast/LSZ263\"\n                ],\n                \"references\": [\n                    {\n                        \"@id\": \"https://api.weather.gov/alerts/urn:oid:2.49.0.1.840.0.e016f252f56054b547b3ac73b3419f6e51da412e.002.2\",\n                        \"identifier\": \"urn:oid:2.49.0.1.840.0.e016f252f56054b547b3ac73b3419f6e51da412e.002.2\",\n                        \"sender\": \"w-nws.webmaster@noaa.gov\",\n                        \"sent\": \"2025-12-03T03:23:00-05:00\"\n                    }\n                ],\n                \"sent\": \"2025-12-03T10:58:00-05:00\",\n                \"effective\": \"2025-12-03T10:58:00-05:00\",\n                \"onset\": \"2025-12-03T16:00:00-05:00\",\n                \"expires\": \"2025-12-03T23:00:00-05:00\",\n                \"ends\": \"2025-12-04T01:00:00-05:00\",\n                \"status\": \"Actual\",\n                \"messageType\": \"Update\",\n                \"category\": \"Met\",\n                \"severity\": \"Moderate\",\n                \"certainty\": \"Likely\",\n                \"urgency\": \"Expected\",\n                \"event\": \"Gale Warning\",\n                \"sender\": \"w-nws.webmaster@noaa.gov\",\n                \"senderName\": \"NWS Marquette MI\",\n                \"headline\": \"Gale Warning issued December 3 at 10:58AM EST until December 4 at 1:00AM EST by NWS Marquette MI\",\n                \"description\": \"* WHAT...For the Gale Warning, northwest winds 25 to 30 kt with\\ngusts up to 35 kt and waves 6 to 9 ft expected. For the Heavy\\nFreezing Spray Warning, heavy freezing spray at a rate of 2 cm\\nper hour or greater expected, and may rapidly accumulate on\\nvessels.\\n\\n* WHERE...Lake Superior from Saxon Harbor WI to Upper Entrance\\nto Portage Canal MI 5NM off shore to the US/Canadian border\\nincluding Isle Royale National Park.\\n\\n* WHEN...For the Gale Warning, from 4 PM this afternoon to 1 AM\\nEST Thursday. For the Heavy Freezing Spray Warning, from 7 PM\\nthis evening to 7 AM EST Thursday.\\n\\n* IMPACTS...Operating a vessel in heavy freezing spray is\\nhazardous. Freezing spray may render mechanical and electronic\\ncomponents inoperative. Rapid ice accretion on decks and\\nsuperstructures may result in a catastrophic loss of\\nstability. Strong winds will cause hazardous waves which could\\ncapsize or damage vessels and reduce visibility.\",\n                \"instruction\": \"Mariners should prepare for dangerous accumulation of ice on\\ntheir vessel. If possible, remain in port, avoid the warning area\\nor conduct mitigation.\\n\\nMariners should alter plans to avoid these hazardous conditions.\\nRemain in port, seek safe harbor, alter course, and/or secure the\\nvessel for hazardous conditions.\",\n                \"response\": \"Avoid\",\n                \"parameters\": {\n                    \"AWIPSidentifier\": [\n                        \"MWWMQT\"\n                    ],\n                    \"WMOidentifier\": [\n                        \"WHUS73 KMQT 031558\"\n                    ],\n                    \"NWSheadline\": [\n                        \"GALE WARNING REMAINS IN EFFECT FROM 4 PM THIS AFTERNOON TO 1 AM EST THURSDAY... ...HEAVY FREEZING SPRAY WARNING REMAINS IN EFFECT FROM 7 PM THIS EVENING TO 7 AM EST THURSDAY\"\n                    ],\n                    \"BLOCKCHANNEL\": [\n                        \"EAS\",\n                        \"NWEM\",\n                        \"CMAS\"\n                    ],\n                    \"VTEC\": [\n                        \"/O.CON.KMQT.GL.W.0057.251203T2100Z-251204T0600Z/\"\n                    ],\n                    \"eventEndingTime\": [\n                        \"2025-12-04T01:00:00-05:00\"\n                    ]\n                },\n                \"scope\": \"Public\",\n                \"code\": \"IPAWSv1.0\",\n                \"language\": \"en-US\",\n                \"web\": \"http://www.weather.gov\",\n                \"eventCode\": {\n                    \"SAME\": [\n                        \"NWS\"\n                    ],\n                    \"NationalWeatherService\": [\n                        \"GLW\"\n                    ]\n                }\n            }\n        },\n        {\n            \"id\": \"https://api.weather.gov/alerts/urn:oid:2.49.0.1.840.0.cfec64fd36b2ac790d0ebe73b8c20f8dfc3ec5cb.002.2\",\n            \"type\": \"Feature\",\n            \"geometry\": null,\n            \"properties\": {\n                \"@id\": \"https://api.weather.gov/alerts/urn:oid:2.49.0.1.840.0.cfec64fd36b2ac790d0ebe73b8c20f8dfc3ec5cb.002.2\",\n                \"@type\": \"wx:Alert\",\n                \"id\": \"urn:oid:2.49.0.1.840.0.cfec64fd36b2ac790d0ebe73b8c20f8dfc3ec5cb.002.2\",\n                \"areaDesc\": \"Lake Superior from Saxon Harbor WI to Upper Entrance to Portage Canal MI 5NM off shore to the US/Canadian border including Isle Royale National Park\",\n                \"geocode\": {\n                    \"SAME\": [\n                        \"091263\"\n                    ],\n                    \"UGC\": [\n                        \"LSZ263\"\n                    ]\n                },\n                \"affectedZones\": [\n                    \"https://api.weather.gov/zones/forecast/LSZ263\"\n                ],\n                \"references\": [\n                    {\n                        \"@id\": \"https://api.weather.gov/alerts/urn:oid:2.49.0.1.840.0.e016f252f56054b547b3ac73b3419f6e51da412e.002.3\",\n                        \"identifier\": \"urn:oid:2.49.0.1.840.0.e016f252f56054b547b3ac73b3419f6e51da412e.002.3\",\n                        \"sender\": \"w-nws.webmaster@noaa.gov\",\n                        \"sent\": \"2025-12-03T03:23:00-05:00\"\n                    }\n                ],\n                \"sent\": \"2025-12-03T10:58:00-05:00\",\n                \"effective\": \"2025-12-03T10:58:00-05:00\",\n                \"onset\": \"2025-12-03T19:00:00-05:00\",\n                \"expires\": \"2025-12-03T23:00:00-05:00\",\n                \"ends\": \"2025-12-04T07:00:00-05:00\",\n                \"status\": \"Actual\",\n                \"messageType\": \"Update\",\n                \"category\": \"Met\",\n                \"severity\": \"Severe\",\n                \"certainty\": \"Likely\",\n                \"urgency\": \"Expected\",\n                \"event\": \"Heavy Freezing Spray Warning\",\n                \"sender\": \"w-nws.webmaster@noaa.gov\",\n                \"senderName\": \"NWS Marquette MI\",\n                \"headline\": \"Heavy Freezing Spray Warning issued December 3 at 10:58AM EST until December 4 at 7:00AM EST by NWS Marquette MI\",\n                \"description\": \"* WHAT...For the Gale Warning, northwest winds 25 to 30 kt with\\ngusts up to 35 kt and waves 6 to 9 ft expected. For the Heavy\\nFreezing Spray Warning, heavy freezing spray at a rate of 2 cm\\nper hour or greater expected, and may rapidly accumulate on\\nvessels.\\n\\n* WHERE...Lake Superior from Saxon Harbor WI to Upper Entrance\\nto Portage Canal MI 5NM off shore to the US/Canadian border\\nincluding Isle Royale National Park.\\n\\n* WHEN...For the Gale Warning, from 4 PM this afternoon to 1 AM\\nEST Thursday. For the Heavy Freezing Spray Warning, from 7 PM\\nthis evening to 7 AM EST Thursday.\\n\\n* IMPACTS...Operating a vessel in heavy freezing spray is\\nhazardous. Freezing spray may render mechanical and electronic\\ncomponents inoperative. Rapid ice accretion on decks and\\nsuperstructures may result in a catastrophic loss of\\nstability. Strong winds will cause hazardous waves which could\\ncapsize or damage vessels and reduce visibility.\",\n                \"instruction\": \"Mariners should prepare for dangerous accumulation of ice on\\ntheir vessel. If possible, remain in port, avoid the warning area\\nor conduct mitigation.\\n\\nMariners should alter plans to avoid these hazardous conditions.\\nRemain in port, seek safe harbor, alter course, and/or secure the\\nvessel for hazardous conditions.\",\n                \"response\": \"Avoid\",\n                \"parameters\": {\n                    \"AWIPSidentifier\": [\n                        \"MWWMQT\"\n                    ],\n                    \"WMOidentifier\": [\n                        \"WHUS73 KMQT 031558\"\n                    ],\n                    \"NWSheadline\": [\n                        \"GALE WARNING REMAINS IN EFFECT FROM 4 PM THIS AFTERNOON TO 1 AM EST THURSDAY... ...HEAVY FREEZING SPRAY WARNING REMAINS IN EFFECT FROM 7 PM THIS EVENING TO 7 AM EST THURSDAY\"\n                    ],\n                    \"BLOCKCHANNEL\": [\n                        \"EAS\",\n                        \"NWEM\",\n                        \"CMAS\"\n                    ],\n                    \"VTEC\": [\n                        \"/O.CON.KMQT.UP.W.0017.251204T0000Z-251204T1200Z/\"\n                    ],\n                    \"eventEndingTime\": [\n                        \"2025-12-04T07:00:00-05:00\"\n                    ]\n                },\n                \"scope\": \"Public\",\n                \"code\": \"IPAWSv1.0\",\n                \"language\": \"en-US\",\n                \"web\": \"http://www.weather.gov\",\n                \"eventCode\": {\n                    \"SAME\": [\n                        \"NWS\"\n                    ],\n                    \"NationalWeatherService\": [\n                        \"UPW\"\n                    ]\n                }\n            }\n        },\n        {\n            \"id\": \"https://api.weather.gov/alerts/urn:oid:2.49.0.1.840.0.cfec64fd36b2ac790d0ebe73b8c20f8dfc3ec5cb.004.1\",\n            \"type\": \"Feature\",\n            \"geometry\": null,\n            \"properties\": {\n                \"@id\": \"https://api.weather.gov/alerts/urn:oid:2.49.0.1.840.0.cfec64fd36b2ac790d0ebe73b8c20f8dfc3ec5cb.004.1\",\n                \"@type\": \"wx:Alert\",\n                \"id\": \"urn:oid:2.49.0.1.840.0.cfec64fd36b2ac790d0ebe73b8c20f8dfc3ec5cb.004.1\",\n                \"areaDesc\": \"Ontonagon to Upper Entrance of Portage Canal MI\",\n                \"geocode\": {\n                    \"SAME\": [\n                        \"091242\"\n                    ],\n                    \"UGC\": [\n                        \"LSZ242\"\n                    ]\n                },\n                \"affectedZones\": [\n                    \"https://api.weather.gov/zones/forecast/LSZ242\"\n                ],\n                \"references\": [\n                    {\n                        \"@id\": \"https://api.weather.gov/alerts/urn:oid:2.49.0.1.840.0.e016f252f56054b547b3ac73b3419f6e51da412e.005.1\",\n                        \"identifier\": \"urn:oid:2.49.0.1.840.0.e016f252f56054b547b3ac73b3419f6e51da412e.005.1\",\n                        \"sender\": \"w-nws.webmaster@noaa.gov\",\n                        \"sent\": \"2025-12-03T03:23:00-05:00\"\n                    }\n                ],\n                \"sent\": \"2025-12-03T10:58:00-05:00\",\n                \"effective\": \"2025-12-03T10:58:00-05:00\",\n                \"onset\": \"2025-12-03T10:58:00-05:00\",\n                \"expires\": \"2025-12-03T23:00:00-05:00\",\n                \"ends\": \"2025-12-03T16:00:00-05:00\",\n                \"status\": \"Actual\",\n                \"messageType\": \"Update\",\n                \"category\": \"Met\",\n                \"severity\": \"Minor\",\n                \"certainty\": \"Likely\",\n                \"urgency\": \"Expected\",\n                \"event\": \"Small Craft Advisory\",\n                \"sender\": \"w-nws.webmaster@noaa.gov\",\n                \"senderName\": \"NWS Marquette MI\",\n                \"headline\": \"Small Craft Advisory issued December 3 at 10:58AM EST until December 3 at 4:00PM EST by NWS Marquette MI\",\n                \"description\": \"* WHAT...For the Small Craft Advisory, northwest winds 20 to 25\\nkt with gusts up to 30 kt and waves 6 to 8 ft occurring. For\\nthe Gale Warning, northwest winds 20 to 30 kt with gusts up to\\n35 kt and waves 7 to 10 ft expected.\\n\\n* WHERE...Ontonagon to Upper Entrance of Portage Canal MI.\\n\\n* WHEN...For the Small Craft Advisory, until 4 PM EST this\\nafternoon. For the Gale Warning, from 4 PM this afternoon to 1\\nAM EST Thursday.\\n\\n* IMPACTS...Strong winds will cause hazardous waves which could\\ncapsize or damage vessels and reduce visibility.\",\n                \"instruction\": \"Mariners should alter plans to avoid these hazardous conditions.\\nRemain in port, seek safe harbor, alter course, and/or secure the\\nvessel for hazardous conditions.\",\n                \"response\": \"Avoid\",\n                \"parameters\": {\n                    \"AWIPSidentifier\": [\n                        \"MWWMQT\"\n                    ],\n                    \"WMOidentifier\": [\n                        \"WHUS73 KMQT 031558\"\n                    ],\n                    \"NWSheadline\": [\n                        \"SMALL CRAFT ADVISORY REMAINS IN EFFECT UNTIL 4 PM EST THIS AFTERNOON... ...GALE WARNING REMAINS IN EFFECT FROM 4 PM THIS AFTERNOON TO 1 AM EST THURSDAY\"\n                    ],\n                    \"BLOCKCHANNEL\": [\n                        \"EAS\",\n                        \"NWEM\",\n                        \"CMAS\"\n                    ],\n                    \"VTEC\": [\n                        \"/O.CON.KMQT.SC.Y.0189.000000T0000Z-251203T2100Z/\"\n                    ],\n                    \"eventEndingTime\": [\n                        \"2025-12-03T16:00:00-05:00\"\n                    ],\n                    \"expiredReferences\": [\n                        \"w-nws.webmaster@noaa.gov,urn:oid:2.49.0.1.840.0.012a713e44cf33f321dde7a7dd606454111e7dbb.002.1,2025-12-02T22:29:00-05:00 w-nws.webmaster@noaa.gov,urn:oid:2.49.0.1.840.0.74d44099106d0ecd40f7d2a62c56231069593ff3.002.1,2025-12-02T14:53:00-05:00 w-nws.webmaster@noaa.gov,urn:oid:2.49.0.1.840.0.747dd730e6a8b18ac9024c3c055a74162144c3ca.002.1,2025-12-02T10:16:00-05:00 w-nws.webmaster@noaa.gov,urn:oid:2.49.0.1.840.0.9d4c1194cc60ce916e8ebdf8581f4113872ed30b.004.1,2025-12-02T03:21:00-05:00 w-nws.webmaster@noaa.gov,urn:oid:2.49.0.1.840.0.d5ffeb017540aadaf19635157a70b91df6d81e89.001.1,2025-12-01T21:49:00-05:00 w-nws.webmaster@noaa.gov,urn:oid:2.49.0.1.840.0.8e0b0289dce64624742e3cac5fed8c2c4f749952.002.1,2025-12-01T15:58:00-05:00 w-nws.webmaster@noaa.gov,urn:oid:2.49.0.1.840.0.9640ccec5117294f059360172e22d38a03ea6319.006.1,2025-12-01T04:11:00-05:00 w-nws.webmaster@noaa.gov,urn:oid:2.49.0.1.840.0.23de79288a8bd71c3987db2d986f76797fd24f98.001.1,2025-12-01T10:42:00-05:00 w-nws.webmaster@noaa.gov,urn:oid:2.49.0.1.840.0.18c494f8dc68c05a12cd56404dce20aa1dfb12d2.002.1,2025-11-30T21:45:00-05:00 w-nws.webmaster@noaa.gov,urn:oid:2.49.0.1.840.0.0ad5c4a68d08f65b0607fc842e17888924974e61.011.1,2025-11-30T15:48:00-05:00 w-nws.webmaster@noaa.gov,urn:oid:2.49.0.1.840.0.103974583677970a3922feb9d66c92b0b9baaf14.005.1,2025-11-30T10:13:00-05:00 w-nws.webmaster@noaa.gov,urn:oid:2.49.0.1.840.0.64212445ec6a97c8e20b5def6d9ab5bdf6a06d0b.004.1,2025-11-30T04:03:00-05:00 w-nws.webmaster@noaa.gov,urn:oid:2.49.0.1.840.0.3356f19211b81b977c40acd7064227af2c8fbd5d.005.1,2025-11-29T21:29:00-05:00 w-nws.webmaster@noaa.gov,urn:oid:2.49.0.1.840.0.f4b587dc68145abdc558e51c214a4d8127f7d8ae.007.1,2025-11-29T15:04:00-05:00 w-nws.webmaster@noaa.gov,urn:oid:2.49.0.1.840.0.48388e28bdbd6d89c91bf59026f0a3b43d106c1d.002.1,2025-11-29T10:37:00-05:00 w-nws.webmaster@noaa.gov,urn:oid:2.49.0.1.840.0.29cb1482902120f5ca614c1357b3cb80e86663a4.004.1,2025-11-29T04:38:00-05:00\"\n                    ]\n                },\n                \"scope\": \"Public\",\n                \"code\": \"IPAWSv1.0\",\n                \"language\": \"en-US\",\n                \"web\": \"http://www.weather.gov\",\n                \"eventCode\": {\n                    \"SAME\": [\n                        \"NWS\"\n                    ],\n                    \"NationalWeatherService\": [\n                        \"SCY\"\n                    ]\n                }\n            }\n        },\n        {\n            \"id\": \"https://api.weather.gov/alerts/urn:oid:2.49.0.1.840.0.cfec64fd36b2ac790d0ebe73b8c20f8dfc3ec5cb.001.2\",\n            \"type\": \"Feature\",\n            \"geometry\": null,\n            \"properties\": {\n                \"@id\": \"https://api.weather.gov/alerts/urn:oid:2.49.0.1.840.0.cfec64fd36b2ac790d0ebe73b8c20f8dfc3ec5cb.001.2\",\n                \"@type\": \"wx:Alert\",\n                \"id\": \"urn:oid:2.49.0.1.840.0.cfec64fd36b2ac790d0ebe73b8c20f8dfc3ec5cb.001.2\",\n                \"areaDesc\": \"Eagle River to Manitou Island MI; Lake Superior from Upper Entrance to Portage Canal to Manitou Island MI 5NM off shore to the US/Canadian Border; Lake Superior East of a line from Manitou Island to Marquette MI and West of a line from Grand Marais MI to the US/Canadian Border Beyond 5NM from shore\",\n                \"geocode\": {\n                    \"SAME\": [\n                        \"091244\",\n                        \"091264\",\n                        \"091266\"\n                    ],\n                    \"UGC\": [\n                        \"LSZ244\",\n                        \"LSZ264\",\n                        \"LSZ266\"\n                    ]\n                },\n                \"affectedZones\": [\n                    \"https://api.weather.gov/zones/forecast/LSZ244\",\n                    \"https://api.weather.gov/zones/forecast/LSZ264\",\n                    \"https://api.weather.gov/zones/forecast/LSZ266\"\n                ],\n                \"r
